vi "dialogbox.vi"(10 "?":string) -> (1 "Boolean":bool=TRUE)   [LabVIEW 2018]
panel:
  out "?":string
  in  "OK":bool
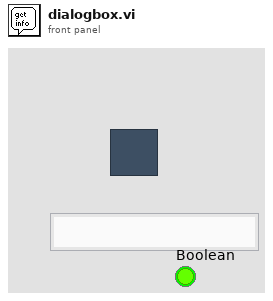
[diagram p1: front panel]
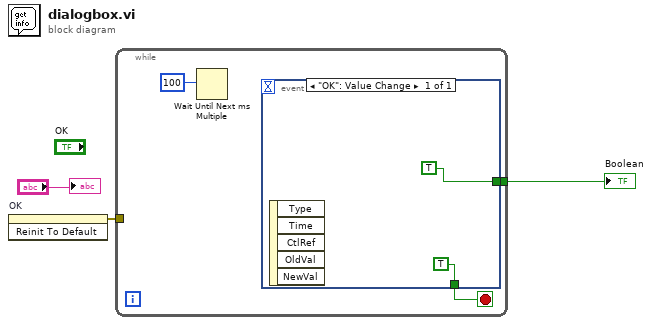
[diagram p0: block diagram]
diagram:
  n1 = invoke on="OK" class="Bool" method="Reinit To Default"() -> (error out=w3:errorcluster)  [unwired: 3 in, 2 out]
  n2 = while {
    tunnel: w3 -> [_]
    tunnel: [w4] -> w2
    stop <- w5 stop-if-true
    n3 = Wait Until Next ms Multiple(millisecond multiple=100) -> ()  [unwired: 1 out]
    n4 = event shown="[0] \"OK\": Value Change" {
      selector: _ -> [_]
      dyn-events: _ -> [_]
      timeout: _ -> [_]
      tunnel: [TRUE] -> w5
      tunnel: [TRUE] -> w4
      event "OK": Value Change {
        n5 = event-data() -> ()  [unwired: 6 out]
      }
    }
  }
  "Boolean" <- w2
  "?" <- "?"
